vi "Array String To Indexed String.vi"(5 "Index [0]":i32, 7 "Array indexing [T]":bool=TRUE, 8 "error in (no error)":errorcluster, 10 "String (RAW)":string, 11 "Registry Object":refnum<class "Carya Config.lvclass">) -> (0 "error out":errorcluster, 2 "String":string, 3 "Registry Object":refnum<class "Carya Config.lvclass">)   [LabVIEW 2013, in "Carya Config.lvclass"]
doc: "Copyright 2018, Carya Automatisering, Wiebe Walstra."
uses:
  Carya Config.lvclass
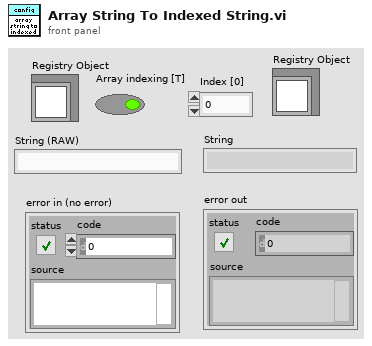
[diagram p1: front panel]
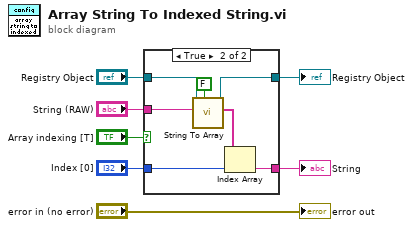
[diagram p0: block diagram]
diagram:
  n1 = case shown="True" "Array indexing [T]" {
    tunnel: [w9 w10] -> w6
    tunnel: "String (RAW)" -> [w9 w16]
    tunnel: "Registry Object" -> [w8 w15]
    tunnel: [w8 w14] -> w2
    tunnel: "Index [0]" -> [_ w11]
    frame False {
    }
    frame True {
      n2 = call-dynamic "String To Array.vi"("Strip Whitespace? [T]"=FALSE, "resulting string"=w16, "Registry Object"=w15) -> ("Array"=w12:string[], "Registry Object"=w14:refnum<class "Carya Config.lvclass">)  [unwired: 6 in, 1 out]
      n3 = Index Array(array=w12, index=w11) -> (element=w10:string)
    }
  }
  "Registry Object" <- w2
  "String" <- w6
  "error out" <- "error in (no error)"
